vi "等待-读写间隔1.vi"(6 "BUSY引用":refnum<vi>, 7 "强制停止？引用":refnum<vi>, 8 "忙时等待？":bool=TRUE, 9 "设置超时(默认-1,单位ms)":i32=-1, 10 "等待字节数(500k)":u32=524288, 11 "VISA资源名i":refnum<visa-resource-name>) -> (0 "超时？":bool, 1 "读取时间s":dbl, 2 "读取字节数":u32=17, 3 "VISA资源名o":refnum<visa-resource-name>)   [LabVIEW 2013]
panel:
  out "读取完毕？":bool
  out ">=字节数？":bool
  out "确认次数？":bool
  in  "停止按钮":bool
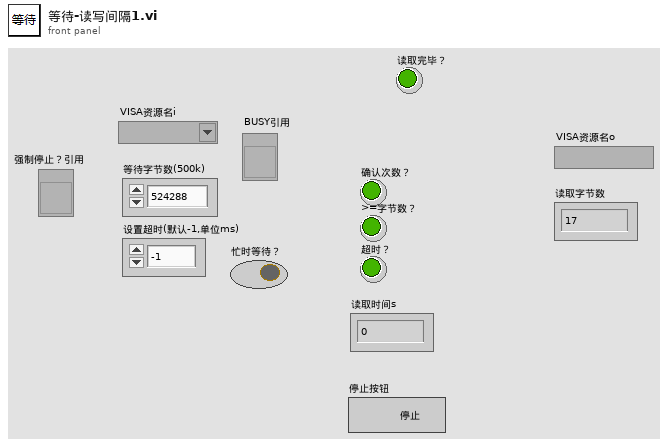
[diagram p1: front panel]
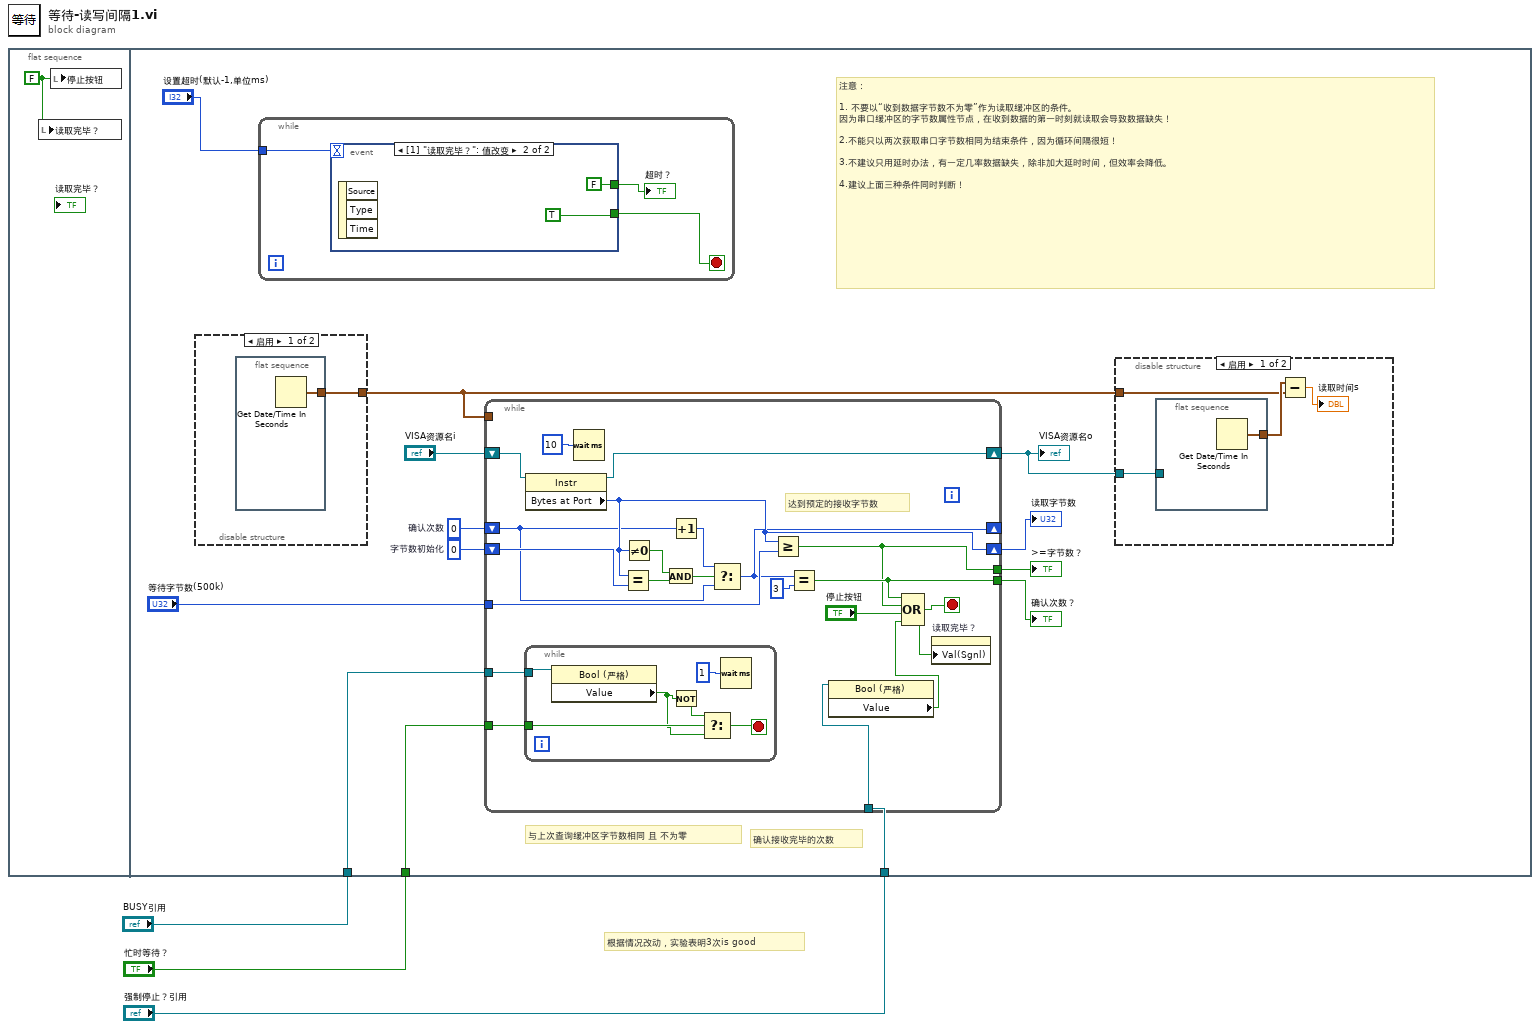
[diagram p0: block diagram]
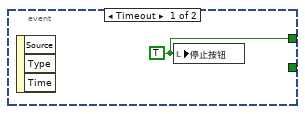
[diagram p2: hidden frame]
diagram:
  # "根据情况改动，实验表明3次is good"
  n1 = flat-sequence {
    tunnel: "BUSY引用" -> [w10]
    tunnel: "忙时等待？" -> [w9]
    tunnel: "强制停止？引用" -> [w8]
    frame #0 {
      w4 = FALSE ("停止按钮")
      n2 = local write "读取完毕？"(w4) -> ()
      n3 = local write "停止按钮"(w4) -> ()
    }
    frame #1 {
      w13 = u32 0  # 确认次数
      w15 = u32 0  # 字节数初始化
      # "确认接收完毕的次数"
      # "与上次查询缓冲区字节数相同 且 不为零"
      # "注意：\n\n1. 不要以“收到数据字节数不为零”作为读取缓冲区的条件。\n因为串口缓冲区的字节数属性节点，在收到数据的第一时刻就读取会导致数据缺失！\n\n2.不能只以两次获取串口字节数相同为结束条件，因为循环间隔很短！\n\n3.不建议只用延时办法，有一定几率数据缺失，除非加大延时时间，但效率会降低。\n\n4.建议上面三种条件同时判断！"
      n4 = disable-structure shown="启用" {
        disable-tunnel: [w29 _] -> w7
        frame Enabled {
          n5 = flat-sequence {
            tunnel: [w30] -> w29
            frame #0 {
              n6 = Get Date/Time In Seconds() -> (seconds since 1Jan1904=w30:timestamp)
            }
          }
        }
        frame Disabled {
        }
      }
      n7 = while {
        tunnel: "设置超时(默认-1,单位ms)" -> [w20]
        stop <- w19 stop-if-true
        n8 = event shown="[1] \"读取完毕？\": 值改变" {
          selector: _ -> [_ _]
          dyn-events: _ -> [_ _]
          timeout: w20 -> [_ _]
          tunnel: [_ TRUE ("读取完毕？ 2")] -> w19
          tunnel: [w21 FALSE ("停止按钮")] -> w18
          event Timeout {
            w21 = TRUE ("停止按钮")
            n9 = event-data() -> ()  [unwired: 1 in, 3 out]
            n10 = local write "停止按钮"(w21) -> ()
          }
          event "读取完毕？": Value Change {
            n11 = event-data() -> ()  [unwired: 1 in, 3 out]
          }
        }
        "超时？" <- w18
      }
      n12 = while {
        shift-right: [w51] -> w6
        shift-left: "VISA资源名i" -> [w49]
        tunnel: "等待字节数(500k)" -> [w48]
        shift-right: [w46] -> w14
        shift-left: w15 -> [w45]
        shift-right: [w42] -> _
        shift-left: w13 -> [w41]
        tunnel: [w38] -> w12
        tunnel: [w37] -> w11
        tunnel: w10 -> [w35]
        tunnel: w9 -> [w34]
        tunnel: w8 -> [w33]
        tunnel: w7 -> [_]
        stop <- w31 stop-if-true
        # "达到预定的接收字节数"
        n13 = while {
          tunnel: w35 -> [w53]
          tunnel: w34 -> [w54]
          stop <- w56 stop-if-true
          n14 = property class="Bool (严格)"(reference=w53) -> ("Value"=w52:bool)  [unwired: 1 in, 2 out]
          n15 = Not(x=w52) -> (.not. x?=w55:bool)
          n16 = Select(t=w55, s=w54, f=w52) -> (s? t:f=w56:bool)
          n17 = Wait (ms)(milliseconds to wait=u32 1 ("等待时间（毫秒）")) -> ()  [unwired: 1 out]
        }
        n18 = property class="Instr"(reference=w49) -> (reference out=w51:refnum<visa-resource-name>, "Bytes at Port"=w46:u32)  [unwired: 1 in, 1 out]
        n19 = Wait (ms)(milliseconds to wait=u32 10 ("等待时间（毫秒）")) -> ()  [unwired: 1 out]
        n20 = Equal?(x=w46, y=w45) -> (x = y?=w40:bool)
        n21 = Not Equal To 0?(x=w46) -> (x != 0?=w47:bool)
        n22 = And(x=w47, y=w40) -> (x .and. y?=w39:bool)
        n23 = Increment(x=w41) -> (x+1=w44:u32)
        n24 = Select(t=w44, s=w39, f=w41) -> (s? t:f=w42:u32)
        n25 = Greater Or Equal?(x=w46, y=w48) -> (x >= y?=w37:bool)
        n26 = Equal?(x=w42, y=u32 3) -> (x = y?=w38:bool)
        n27 = property class="Bool (严格)"(reference=w33) -> ("Value"=w32:bool)  [unwired: 1 in, 2 out]
        n28 = Compound Arithmetic op=OR(w38, w37, "停止按钮", w32) -> (w31:bool)
        n29 = property on="读取完毕？" class="Bool (严格)"("Val(Sgnl)"=w31) -> ()  [unwired: 2 in, 2 out]
      }
      "读取字节数" <- w14
      "VISA资源名o" <- w6
      "确认次数？" <- w12
      ">=字节数？" <- w11
      n30 = disable-structure shown="启用" {
        disable-tunnel: w7 -> [w26 _]
        disable-tunnel: w6 -> [w24 _]
        frame Enabled {
          n31 = flat-sequence {
            tunnel: [w28] -> w27
            tunnel: w24 -> [_]
            frame #0 {
              n32 = Get Date/Time In Seconds() -> (seconds since 1Jan1904=w28:timestamp)
            }
          }
          n33 = Subtract(x=w27, y=w26) -> (x-y=→"读取时间s":dbl)
        }
        frame Disabled {
        }
      }
    }
  }
